vi "Show Control Theme Levels.vi"(10 "VI Refnum":refnum<vi>) -> ()   [LabVIEW 2021]
doc: "This VI will be the user interface function for the Quick Drop action - it will list all controls on the front panel along with their UI Theme Levels and Boolean Types. This will be populated before showing its front panel and will give the user faster access to edit all controls on the front panel.\n\n->If there are any changes made and \"Apply\" is selected, it will apply the updated tags and save the VI\n->If Cancel is selected, the updates made will not be implemented\n\n<b>Code Developed By:</b>\nTechnology Service Corporation\nwww.tsc.com/atcs\n\nDeveloper:\nDaniel Coons"
uses:
  Quick Drop Plugins/TSC Control Theme Application.llb/control info.ctl
  <vilib>/Utility/traverseref.llb/TRef TravTarget.ctl
  <vilib>/Utility/traverseref.llb/VI Scripting - Traverse.lvlib
  user32.dll
panel:
  out "Name of VI":string
  in  "cancel":bool
  in  "apply":bool
  out "header":bool
  in  "control info":T1[](array[typedef]) {"Boolean Type" items=["Undefined", "N/A", "Outline", "No-Outline", "Tonal", "Filled", "Transparent", "FAB", "Elevated"]; "UI Theme Level" items=["Undefined", "N/A", "Primary", "Secondary", "Tertiary", "Error", "Primary Fixed", "Secondary Fixed", "Tertiary Fixed", "Label Only", "No Change"]}
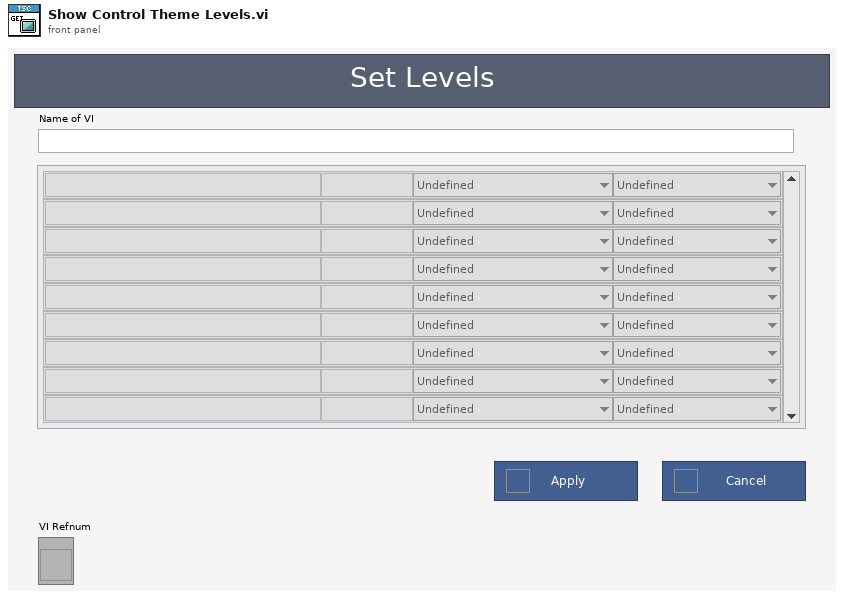
[diagram p1: front panel]
types:
  T1 = typedef "control info.ctl" = cluster{"label":string, "control type":string, "UI Theme Level":u16, "Boolean Type":u16}
  T2 = typedef "TRef TravTarget.ctl" = enum16{"FP", "BD", "Other"}
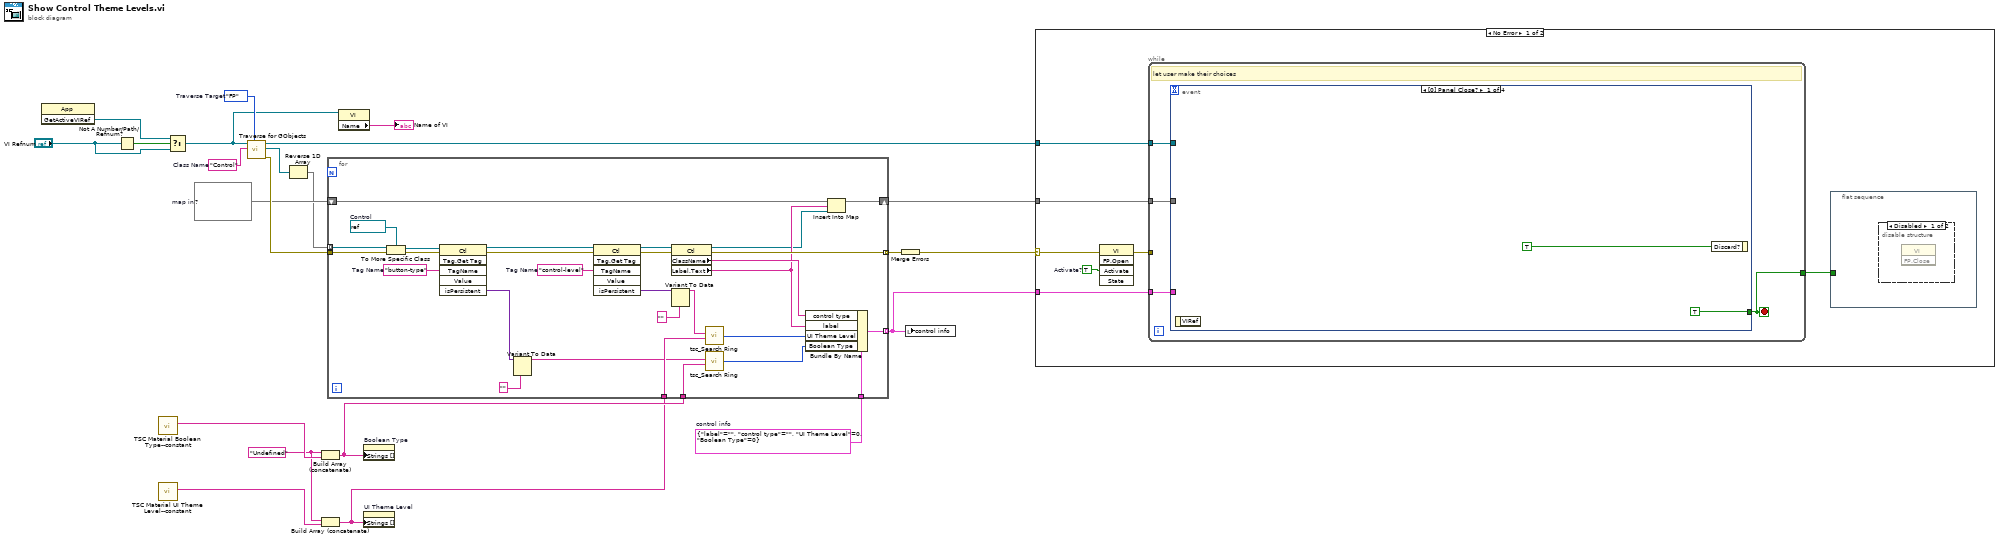
[diagram p0: block diagram]
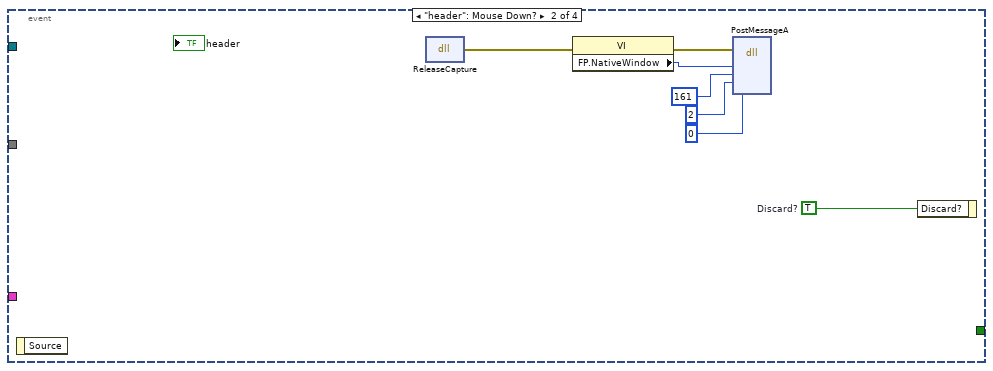
[diagram p3: hidden frame]
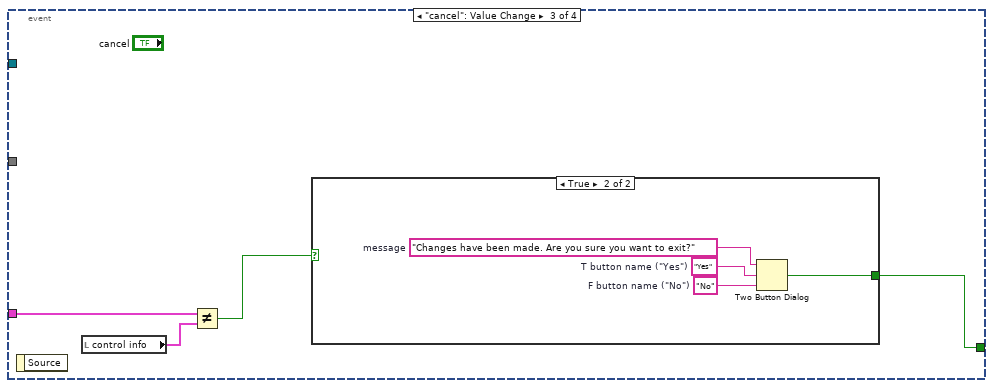
[diagram p4: hidden frame]
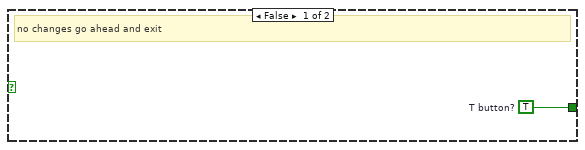
[diagram p5: hidden frame]
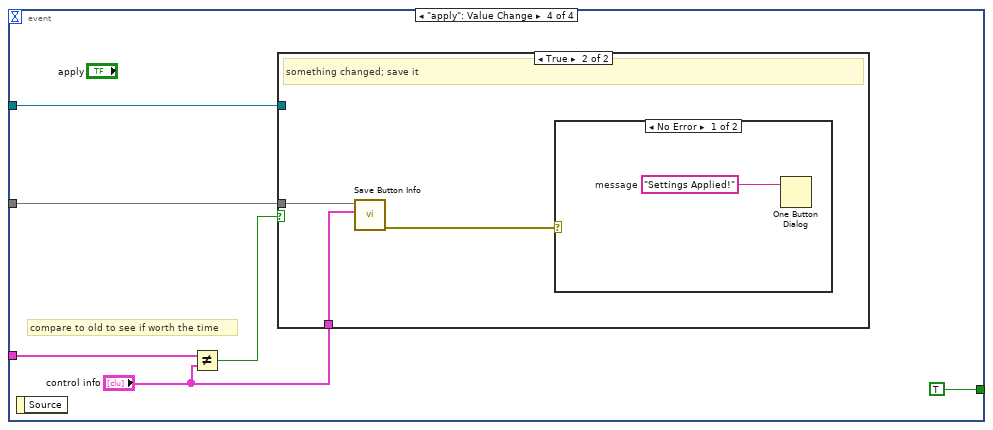
[diagram p6: hidden frame]
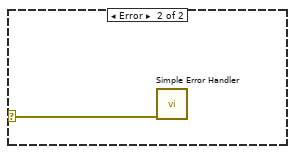
[diagram p8: hidden frame]
diagram:
  w10 = "Undefined"
  w14 = map{string, refnum<vi>} {}  # map in
  w17 = T1 {"label"="", "control type"="", "UI Theme Level"=0, "Boolean Type"=0}  # control info
  w21 = TRef_TravTarget."FP"  # Traverse Target
  w22 = "Control"  # Class Name
  n1 = invoke class="App" method="GetActiveVIRef"() -> ("GetActiveVIRef"=w4:refnum<vi>)  [unwired: 3 in, 2 out]
  n2 = Not A Number/Path/Refnum?(number/path/refnum="VI Refnum") -> (NaN/Path/Refnum?=w5:bool)
  n3 = call "TSC Material Boolean Type--constant.vi"() -> ("boolean types"=w16:string[])  [unwired: 11 in]
  n4 = call "TSC Material UI Theme Level--constant.vi"() -> ("UI theme levels"=w8:string[])  [unwired: 11 in]
  n5 = Select(t=w4, s=w5, f="VI Refnum") -> (s? t:f=w2:refnum<vi>)
  n6 = call <vilib>:"Traverse for GObjects.vi"("Traverse Target"=w21, "Class Name"=w22, "VI Refnum"=w2) -> ("error out"=w19:errorcluster, "References"=w20:refnum<vi>[], "dup VI Refnum"=w11:refnum<vi>)  [unwired: 5 in, 1 out]
  n7 = Reverse 1D Array(array=w20) -> (reversed array=w6:refnum<vi>[])
  n8 = Build Array (concatenate)(w10, w16) -> (w9:string[])
  n9 = Build Array (concatenate)(w10, w8) -> (w7:string[])
  n10 = for {
    tunnel: w6 -> [w38] mode=indexing
    tunnel: w19 -> [w48]
    tunnel: [w41] -> w18 mode=indexing
    tunnel: w17 -> [w35]
    tunnel: w9 -> [w25]
    tunnel: [w33] -> w15 mode=indexing
    tunnel: w7 -> [w28]
    shift-right: [w31] -> w13
    shift-left: w14 -> [w32]
    w36 = refnum<vi> refnum  # Control
    w42 = "control-level"  # Tag Name
    w51 = "button-type"  # Tag Name
    n11 = To More Specific Class(target class=w36, reference=w38, error in=w48) -> (specific class reference=w37:refnum<vi>, error out=w39:errorcluster)
    n12 = invoke class="Ctl" method="Tag.Get Tag"(reference=w37, error in=w39, "TagName"=w51) -> (reference out=w45:refnum<vi>, error out=w47:errorcluster, "isPersistent"=w50:variant)  [unwired: 3 in, 3 out]
    n13 = Variant To Data(type="", Variant=w50) -> (data=w24:string)  [unwired: 1 in, 1 out]
    n14 = invoke class="Ctl" method="Tag.Get Tag"(reference=w45, error in=w47, "TagName"=w42) -> (reference out=w40:refnum<vi>, error out=w46:errorcluster, "isPersistent"=w43:variant)  [unwired: 3 in, 3 out]
    n15 = property class="Ctl"(reference=w40, error in=w46) -> (reference out=w29:refnum<vi>, error out=w41:errorcluster, "ClassName"=w34:string, "Label.Text"=w30:string)
    n16 = Variant To Data(type="", Variant=w43) -> (data=w27:string)  [unwired: 1 in, 1 out]
    n17 = call "tsc_Search Ring.vi"("Values"=w28, "Search Item"=w27) -> ("Index"=w26:u16)  [unwired: 2 in]
    n18 = call "tsc_Search Ring.vi"("Values"=w25, "Search Item"=w24) -> ("Index"=w23:u16)  [unwired: 2 in]
    n19 = Bundle By Name(cluster=w35, "control type"=w34, "label"=w30, "UI Theme Level"=w26, "Boolean Type"=w23) -> (w33:T1)
    n20 = Insert Into Map(map in=w32, key=w30, value=w29) -> (map out=w31:map{string, refnum<vi>})  [unwired: 2 out]
  }
  n21 = property class="VI"(reference=w2) -> ("Name"=→"Name of VI":string)  [unwired: 1 in, 2 out]
  n22 = property on="Boolean Type" class="Ring (strict)"("Strings []"=w9) -> ()  [unwired: 2 in, 2 out]
  n23 = property on="UI Theme Level" class="Ring (strict)"("Strings []"=w7) -> ()  [unwired: 2 in, 2 out]
  n24 = Merge Errors(w18) -> (w12:errorcluster)
  n25 = local write "control info"(w15) -> ()
  n26 = case shown="No Error" w12 {
    selector: w12 -> [w56 _]
    tunnel: w15 -> [w58 _]
    tunnel: w13 -> [w57 _]
    tunnel: w11 -> [w52 _]
    frame No Error {
      w55 = TRUE  # Activate?
      n27 = invoke class="VI" method="FP.Open"(error in=w56, "Activate"=w55) -> (error out=w54:errorcluster)  [unwired: 3 in, 4 out]
      n28 = while {
        tunnel: w58 -> [w62]
        tunnel: w57 -> [w61]
        tunnel: w54 -> [_]
        tunnel: w52 -> [w60]
        tunnel: [w59] -> w53
        stop <- w59 stop-if-true
        # "let user make their choices"
        n29 = event shown="[0] Panel Close?" {
          selector: _ -> [_ _ _ _]
          dyn-events: _ -> [_ _ _ _]
          timeout: _ -> [_ _ _ _]
          tunnel: [TRUE _ w72 TRUE] -> w59
          tunnel: w62 -> [_ _ w75 w85]
          tunnel: w61 -> [_ _ _ w84]
          tunnel: w60 -> [_ _ _ w81]
          event Panel Close? {
            n30 = event-data() -> ()  [unwired: 1 in, 1 out]
            n31 = event-data("Discard?"=TRUE) -> ()  [unwired: 1 in, 1 out]
          }
          event "header": Mouse Down? {
            w65 = TRUE  # Discard?
            n32 = event-data() -> ()  [unwired: 1 in, 1 out]
            n33 = dll-call lib="user32.dll" fn="ReleaseCapture"() -> (error out=w68:errorcluster)  [unwired: 4 in, 1 out]
            n34 = property class="VI"(error in=w68) -> (error out=w67:errorcluster, "FP.NativeWindow"=w66:u64)  [unwired: 1 in, 1 out]
            n35 = dll-call lib="user32.dll" fn="PostMessageA"(error in=w67, "hWnd"=w66, "Msg"=161, "wParam"=2, "lParam"=0) -> ()  [unwired: 7 in, 2 out]
            n36 = event-data("Discard?"=w65) -> ()  [unwired: 1 in, 1 out]
          }
          event "cancel": Value Change {
            n37 = event-data() -> ()  [unwired: 1 in, 1 out]
            n38 = local read "control info"() -> (w74:T1[])
            n39 = Not Equal?(x=w75, y=w74) -> (x != y?=w73:bool)
            n40 = case shown="True" w73 {
              tunnel: [w76 w77] -> w72
              frame False {
                w76 = TRUE  # T button?
                # "no changes go ahead and exit"
              }
              frame True {
                w80 = "No"  # F button name ("No")
                w79 = "Yes"  # T button name ("Yes")
                w78 = "Changes have been made. Are you sure you want to exit?"  # message
                n41 = Two Button Dialog(message=w78, 1:w80, 2:w79) -> (T button?=w77:bool)
              }
            }
          }
          event "apply": Value Change {
            # "compare to old to see if worth the time"
            n42 = event-data() -> ()  [unwired: 1 in, 1 out]
            n43 = Not Equal?(x=w85, y="control info") -> (x != y?=w82:bool)
            n44 = case shown="True" w82 {
              tunnel: w84 -> [_ w89]
              tunnel: "control info" -> [_ w88]
              tunnel: w81 -> [_ _]
              frame False {
              }
              frame True {
                # "something changed; save it"
                n45 = call "Save Button Info.vi"("control info"=w88, "map in"=w89) -> ("error out"=w87:errorcluster)  [unwired: 9 in]
                n46 = case shown="No Error" w87 {
                  selector: w87 -> [_ w91]
                  frame No Error {
                    w90 = "Settings Applied!"  # message
                    n47 = One Button Dialog(message=w90) -> ()  [unwired: 1 in, 1 out]
                  }
                  frame Error {
                    n48 = call <vilib>:"Simple Error Handler.vi"("error in (no error)"=w91) -> ()  [unwired: 4 in, 5 out]
                  }
                }
              }
            }
          }
        }
      }
      n49 = flat-sequence {
        tunnel: w53 -> [_]
        frame #0 {
          n50 = disable-structure shown="Disabled" {
            frame Disabled {
              n51 = invoke class="VI" method="FP.Close"() -> ()  [unwired: 3 in, 3 out]
            }
            frame Enabled {
            }
          }
        }
      }
    }
    frame Error {
    }
  }
